vi "SETParametersToSPCdata.vi"(8 "ErrorIn":errorcluster, 10 "setFile":path=path "X:/Jannis/Abgleich/150-n scanin.set", 11 "SPCdataIn":T1={"base_adr"=0, "init"=0, "cfd_limit_low"=0.0, "cfd_limit_high"=0.0, "cfd_zc_level"=0.0, "cfd_holdoff"=0.0, "sync_zc_level"=0.0, "sync_holdoff"=0.0, "sync_threshold"=0.0, "tac_range"=0.0, "sync_freq_div"=0, "tac_gain"=0, "tac_offset"=0.0, "tac_limit_low"=0.0, "tac_limit_high"=0.0, "adc_resolution"=12, "ext_latch_delay"=0, "collect_time"=0.0, "display_time"=0.0, "repeat_time"=0.0, "stop_on_time"=0, "stop_on_ovfl"=0, "dither_range"=0, "count_incr"=0, "mem_bank"=0, "dead_time_comp"=0, "scan_control"=0, "routing_mode"=0, "tac_enable_hold"=0.0, "pci_card_no"=0, "mode"=0, "scan_size_x"=0, "scan_size_y"=0, "scan_rout_x"=0, "scan_rout_y"=0, "scan_flyback"=0, "scan_borders"=0, "scan_polarity"=0, "pixel_clock"=0, "line_compression"=0, "trigger"=0, "pixel_time"=0.0, "ext_pixclk_div"=0, "rate_count_time"=0.0, "macro_time_clk"=0, "add_select"=0, "test_eep"=0, "adc_zoom"=0, "img_size_x"=0, "img_size_y"=0, "img_rout_x"=0, "img_rout_y"=0, "xy_gain"=0, "master_clock"=0, "adc_sample_delay"=0, "detector_type"=0, "chan_enable"=0, "chan_slope"=0, "chan_spec_no"=0, "tdc_control"=0, "tdc_offset1"=0.0, "tdc_offset2"=0.0, "tdc_offset3"=0.0, "tdc_offset4"=0.0, "future_reserve1"=0, "future_reserve2"=0, "future_reserve3"=0, "future_reserve4"=0, "future_reserve5"=0, "future_reserve6"=0, "future_reserve7"=0}) -> (0 "ErrorOut":errorcluster, 3 "SPCdataOut":T1={"base_adr"=0, "init"=0, "cfd_limit_low"=0.0, "cfd_limit_high"=0.0, "cfd_zc_level"=0.0, "cfd_holdoff"=0.0, "sync_zc_level"=0.0, "sync_holdoff"=0.0, "sync_threshold"=0.0, "tac_range"=0.0, "sync_freq_div"=0, "tac_gain"=0, "tac_offset"=0.0, "tac_limit_low"=0.0, "tac_limit_high"=0.0, "adc_resolution"=12, "ext_latch_delay"=0, "collect_time"=0.0, "display_time"=0.0, "repeat_time"=0.0, "stop_on_time"=0, "stop_on_ovfl"=0, "dither_range"=0, "count_incr"=0, "mem_bank"=0, "dead_time_comp"=0, "scan_control"=0, "routing_mode"=0, "tac_enable_hold"=0.0, "pci_card_no"=0, "mode"=0, "scan_size_x"=0, "scan_size_y"=0, "scan_rout_x"=0, "scan_rout_y"=0, "scan_flyback"=0, "scan_borders"=0, "scan_polarity"=0, "pixel_clock"=0, "line_compression"=0, "trigger"=0, "pixel_time"=0.0, "ext_pixclk_div"=0, "rate_count_time"=0.0, "macro_time_clk"=0, "add_select"=0, "test_eep"=0, "adc_zoom"=0, "img_size_x"=0, "img_size_y"=0, "img_rout_x"=0, "img_rout_y"=0, "xy_gain"=0, "master_clock"=0, "adc_sample_delay"=0, "detector_type"=0, "chan_enable"=0, "chan_slope"=0, "chan_spec_no"=0, "tdc_control"=0, "tdc_offset1"=0.0, "tdc_offset2"=0.0, "tdc_offset3"=0.0, "tdc_offset4"=0.0, "future_reserve1"=0, "future_reserve2"=0, "future_reserve3"=0, "future_reserve4"=0, "future_reserve5"=0, "future_reserve6"=0, "future_reserve7"=0}, 5 "ActiveModule":string[](array[string]))   [LabVIEW 2019]
doc: "This VI aids to read a full set of system parameters from a .set-file or the header of a .sdt into the SPCdata cluster. Usefull when wanting to copy all parameters established in SPCM.exe to the LV-environment.\nNote, that some parameters like <b>mode</b> are not mapped. To correctly set these parameters use SPC_set- and get_parameters.vi before calling this VI."
uses:
  SPC_Controls/Systparm_Kewords.ctl
  SPC_Controls/SPCdata.ctl
panel:
  out "String":string
  in  "Systparm_Keywords":T2
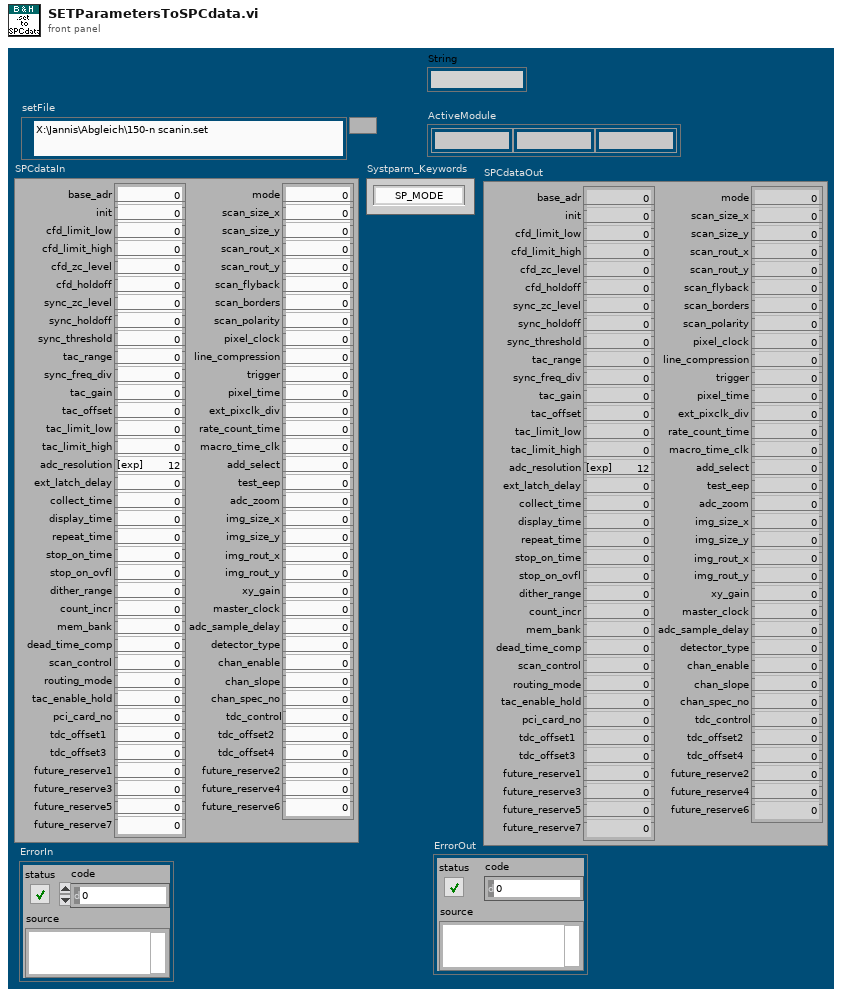
[diagram p1: front panel]
types:
  T1 = typedef "SPCdata.ctl" = cluster{"base_adr":u16, "init":i16, "cfd_limit_low":sgl, "cfd_limit_high":sgl, "cfd_zc_level":sgl, "cfd_holdoff":sgl, "sync_zc_level":sgl, "sync_holdoff":sgl, "sync_threshold":sgl, "tac_range":sgl, "sync_freq_div":i16, "tac_gain":i16, "tac_offset":sgl, "tac_limit_low":sgl, "tac_limit_high":sgl, "adc_resolution":i16, "ext_latch_delay":i16, "collect_time":sgl, "display_time":sgl, "repeat_time":sgl, "stop_on_time":i16, "stop_on_ovfl":i16, "dither_range":i16, "count_incr":i16, "mem_bank":i16, "dead_time_comp":i16, "scan_control":u16, "routing_mode":u16, "tac_enable_hold":sgl, "pci_card_no":i16, "mode":u16, "scan_size_x":u32, "scan_size_y":u32, "scan_rout_x":u32, "scan_rout_y":u32, "scan_flyback":u32, "scan_borders":u32, "scan_polarity":u16, "pixel_clock":u16, "line_compression":u16, "trigger":u16, "pixel_time":sgl, "ext_pixclk_div":u32, "rate_count_time":sgl, "macro_time_clk":i16, "add_select":i16, "test_eep":i16, "adc_zoom":i16, "img_size_x":u32, "img_size_y":u32, "img_rout_x":u32, "img_rout_y":u32, "xy_gain":i16, "master_clock":i16, "adc_sample_delay":i16, "detector_type":i16, "chan_enable":u32, "chan_slope":u32, "chan_spec_no":u32, "tdc_control":u32, "tdc_offset1":sgl, "tdc_offset2":sgl, "tdc_offset3":sgl, "tdc_offset4":sgl, "future_reserve1":u64, "future_reserve2":u64, "future_reserve3":u64, "future_reserve4":u64, "future_reserve5":u64, "future_reserve6":u64, "future_reserve7":u64}
  T2 = typedef "Systparm_Kewords.ctl" = enum16{"SP_MODE", "SP_CFD_LL", "SP_CFD_LH", "SP_CFD_ZC", "SP_CFD_HF", "SP_SYN_ZC", "SP_SYN_FD", "SP_SYN_FQ", "SP_SYN_HF", "SP_TAC_R", "SP_TAC_G", "SP_TAC_OF", "SP_TAC_LL", "SP_TAC_LH", "SP_TAC_TC", "SP_TAC_TD", "SP_ADC_RE", "SP_EAL_DE", "SP_NCX", "SP_NCY", "SP_PAGE", "SP_COL_T", "SP_REP_T", "SP_DIS_T", "SP_REPEAT", "SP_STOPT", "SP_OVERFL", "SP_WL_STA", "SP_WL_STO", "SP_WL_STE", "SP_EXTST", "SP_STEPS", "SP_OFFSET", "SP_YWIN_N", "SP_XWIN_N", "SP_TWIN_N", "SP_X_EQU", "SP_Y_EQU", "SP_T_EQU", "SP_DITH", "SP_EN_INT", "SP_INCR", "SP_DAES", "SP_SPE_FN", "SP_CYCLES", "SP_DAEC", "SP_MEM_BANK", "SP_DTCOMP", "SP_SCF", "SP_POL_L", "SP_POL_F", "SP_PIX", "SP_LDIV", "SP_ACCUM", "SP_ROUT", "SP_TAC_EH", "SP_DLIM", "SP_PHOT_F", "SP_EN_DLIM", "SP_PH_BUF", "SP_FLB_Y", "SP_FLB_X", "SP_BORD_U", "SP_BORD_L", "SP_POL_P", "SP_PIX_T", "SP_PIX_CLK", "SP_TRIGGER", "SP_SCAN_X", "SP_SCAN_Y", "SP_SCAN_RX", "SP_SCAN_RY", "SP_FIF_TYP", "SP_EPX_DIV", "SP_MTCLK", "SP_ADD_SEL", "SP_SXWIN_N", "SP_SYWIN_N", "SP_SX_EQU", "SP_SY_EQU", "SP_ASAVE", "SP_ADC_ZOOM", "SP_FIF_FNO", "SP_FCYCLES", "SP_XY_GAIN", "SP_IMG_X", "SP_IMG_Y", "SP_IMG_RX", "SP_IMG_RY", "SP_MST_CLK", "SP_ADC_DE", "SP_DET_TYP", "SP_X_AXIS", "SP_CH_EN", "SP_CH_SL", "SP_CH_F1", "SP_CH_F2"}
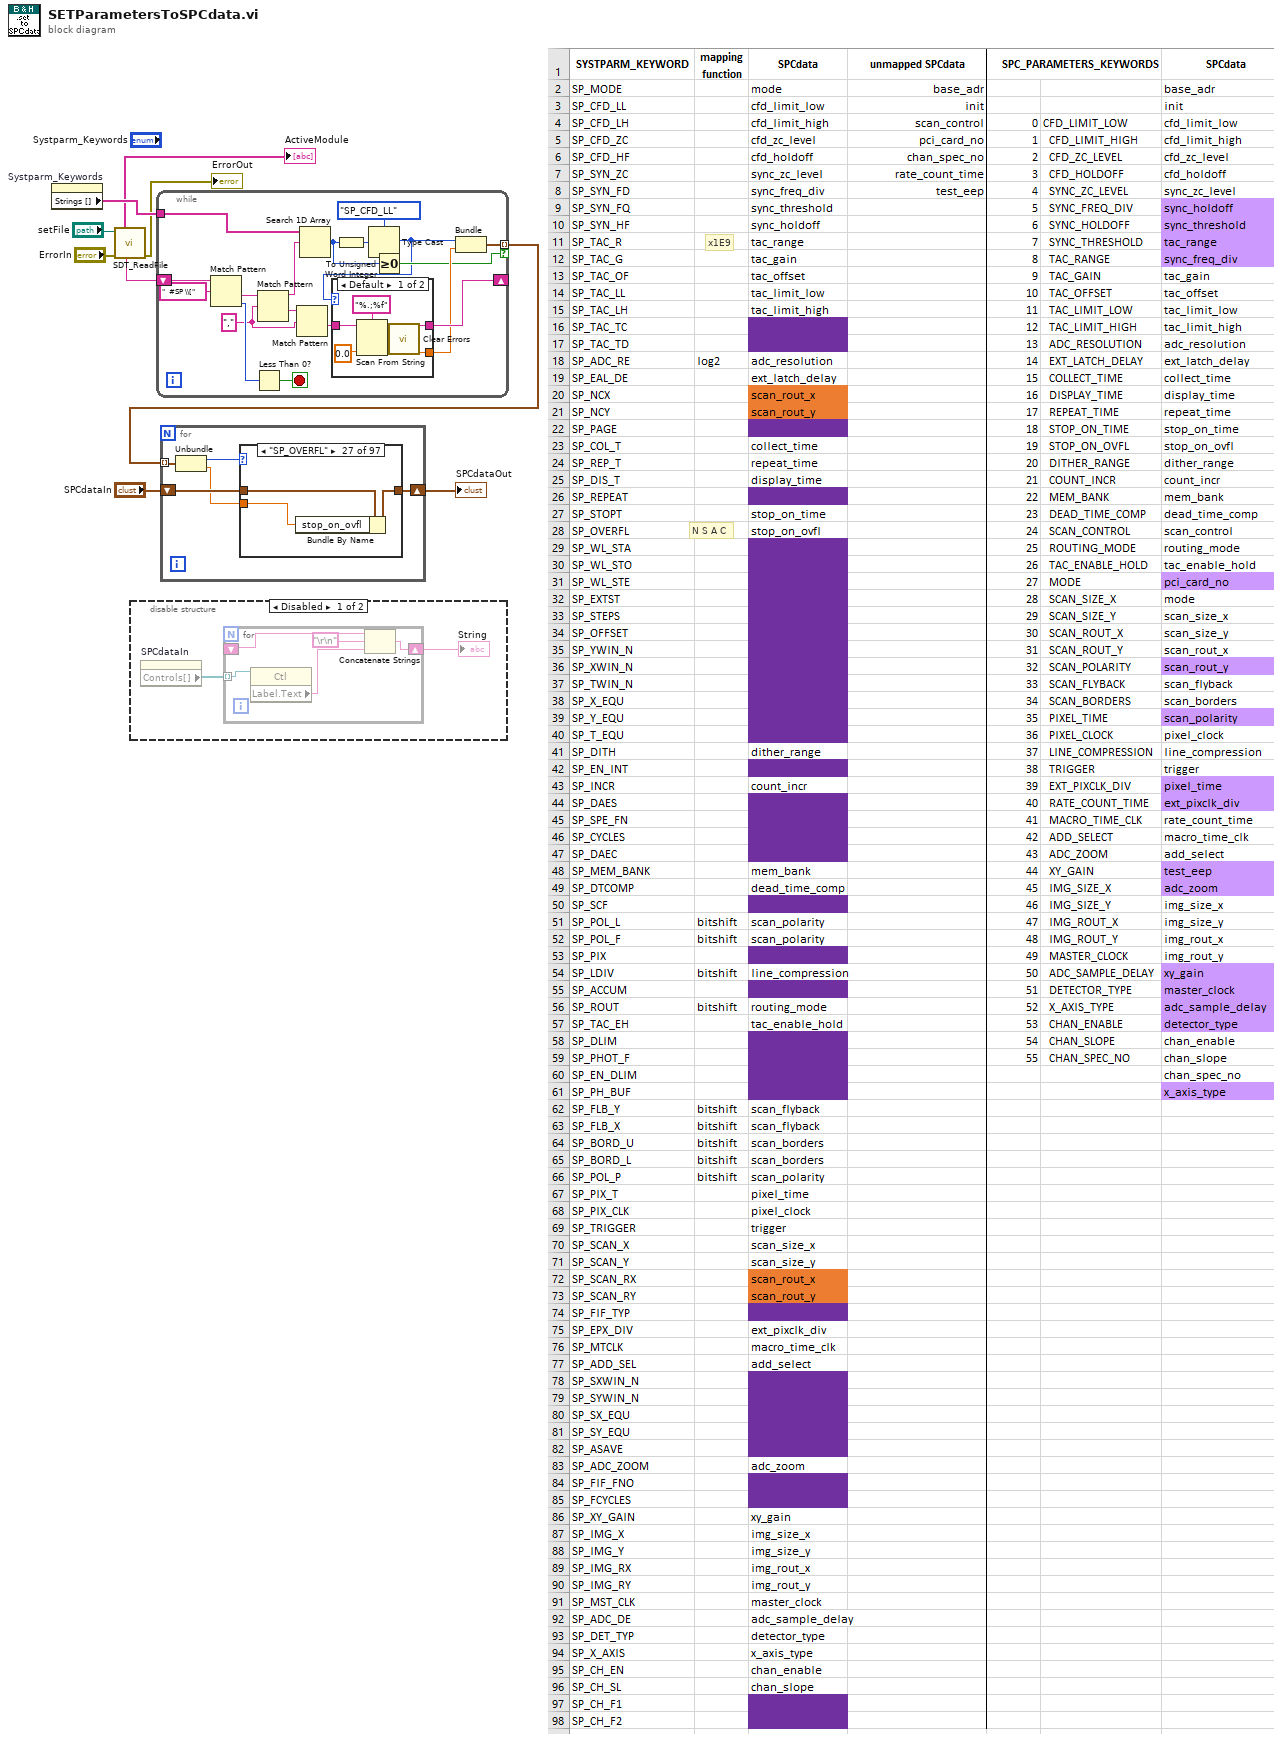
[diagram p0: block diagram]
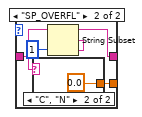
[diagram p2: hidden frame]
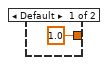
[diagram p3: hidden frame]
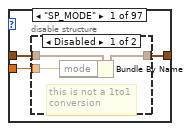
[diagram p5: hidden frame]
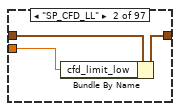
[diagram p7: hidden frame]
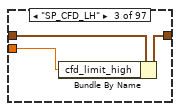
[diagram p8: hidden frame]
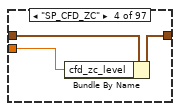
[diagram p9: hidden frame]
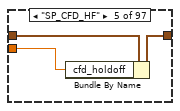
[diagram p10: hidden frame]
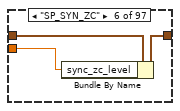
[diagram p11: hidden frame]
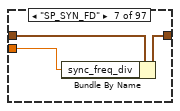
[diagram p12: hidden frame]
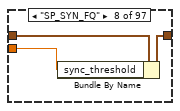
[diagram p13: hidden frame]
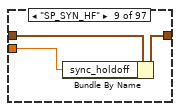
[diagram p14: hidden frame]
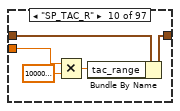
[diagram p15: hidden frame]
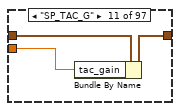
[diagram p16: hidden frame]
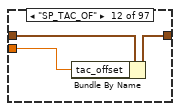
[diagram p17: hidden frame]
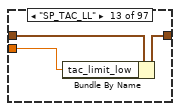
[diagram p18: hidden frame]
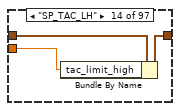
[diagram p19: hidden frame]
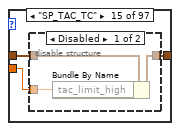
[diagram p20: hidden frame]
diagram:
  # "N S A C"
  # "x1E9"
  n1 = property on="Systparm_Keywords" class="Enum (strict)"() -> ("Strings []"=w5:string[])  [unwired: 2 in, 2 out]
  n2 = call "SDT_ReadFile.vi"("error in"="ErrorIn", "sdtFile"="setFile") -> ("error out"=→"ErrorOut":errorcluster, "SetUp"=w6:string, "ActiveModule"=→"ActiveModule":string[])  [unwired: 2 in, 5 out]
  n3 = disable-structure shown="Disabled" {
    frame Disabled {
      n4 = property on="SPCdataIn" class="Clust (strict)"() -> ("Controls[]"=w11:refnum<vi>[])  [unwired: 2 in, 2 out]
      n5 = for {
        tunnel: w11 -> [w16] mode=indexing
        shift-right: [w14] -> w10
        shift-left: _ -> [w13]
        n6 = property class="Ctl"(reference=w16) -> ("Label.Text"=w15:string)  [unwired: 1 in, 2 out]
        n7 = Concatenate Strings(w13, "\r\n", w15) -> (w14:string)
      }
      "String" <- w10
    }
    frame Enabled {
    }
  }
  n8 = while {
    shift-right: [w26] -> _
    shift-left: w6 -> [w34]
    tunnel: w5 -> [w24]
    tunnel: [w21] -> w4 mode=indexing if=w19
    stop <- w31 stop-if-true
    w28 = "," ("regular expression")
    n9 = Match Pattern(string=w34, regular expression="  #SP \\[") -> (after substring=w32:string, offset past match=w30:i32)  [unwired: 1 in, 2 out]
    n10 = Less Than 0?(x=w30) -> (x < 0?=w31:bool)
    n11 = Match Pattern(string=w32, regular expression=w28) -> (before substring=w25:string, after substring=w29:string)  [unwired: 1 in, 2 out]
    n12 = Match Pattern(string=w29, regular expression=w28) -> (after substring=w27:string)  [unwired: 1 in, 3 out]
    n13 = Search 1D Array(1D array=w24, element=w25) -> (index of element=w20:i32)  [unwired: 1 in]
    n14 = To Unsigned Word Integer(number=w20) -> (unsigned 16bit integer=w18:u16)
    n15 = Type Cast(type=Systparm_Kewords."SP_CFD_LL" ("Systparm_Keywords"), x=w18) -> (*(type *) &x=w17:T2)
    n16 = case shown="Default" w17 {
      tunnel: w27 -> [w40 w42]
      tunnel: [w37 w42] -> w26
      tunnel: [w36 w41] -> w22
      frame Default {
        n17 = Scan From String(format string="%.;%f", input string=w40, default 1=sgl 0.0 ("Value")) -> (remaining string=w37:string, error out=w35:errorcluster, output 1=w36:sgl)  [unwired: 2 in, 1 out]
        n18 = call <vilib>:"Clear Errors.vi"("error in (no error)"=w35) -> ()  [unwired: 5 in, 2 out]
      }
      frame "SP_OVERFL" {
        n19 = String Subset(string=w42, length (rest)=1 ("length (rest)")) -> (substring=w43:string)  [unwired: 1 in]
        n20 = case shown="\"C\", \"N\"" w43 {
          tunnel: [sgl 1.0 ("Value") sgl 0.0 ("Value")] -> w41
          frame Default {
          }
          frame "C", "N" {
          }
        }
      }
    }
    n21 = Greater Or Equal To 0?(x=w20) -> (x >= 0?=w19:bool)
    n22 = Bundle("Systparm_Keywords"=w17, "Value"=w22) -> (w21:cluster{"Systparm_Keywords":T2, "Value":sgl})  [unwired: 1 in]
  }
  n23 = for {
    shift-right: [w50] -> w8
    shift-left: "SPCdataIn" -> [w51]
    tunnel: w4 -> [w49] mode=indexing
    n24 = Unbundle(w49) -> ("Systparm_Keywords"=w48:T2, "Value"=w47:sgl)
    n25 = case shown="\"SP_OVERFL\"" w48 {
      tunnel: w51 -> [w53 w61 w64 w67 w70 w73 w76 w79 w82 w87 w90 w93 w96 w99 w102 w109 w117 w120 w123 w126 w129 w136 w139 w142 w145 w152 w155 w158 w165 w172 w179 w186 w193 w200 w207 w214 w221 w228 w235 w242 w245 w252 w255 w262 w269 w276 w283 w286 w289 w300 w310 w314 w323 w326 w335 w338 w341 w348 w355 w362 w374 w381 w390 w397 w407 w410 w413 w416 w419 w422 w425 w428 w431 w438 w441 w444 w447 w454 w461 w468 w475 w482 w485 w492 w499 w502 w505 w508 w511 w514 w517 w520 w523 w526 w529 w532 w539]
      tunnel: [w54 w60 w63 w66 w69 w72 w75 w78 w81 w86 w89 w92 w95 w98 w101 w108 w116 w119 w122 w125 w128 w135 w138 w141 w144 w151 w154 w157 w164 w171 w178 w185 w192 w199 w206 w213 w220 w227 w234 w241 w244 w251 w254 w261 w268 w275 w282 w285 w288 w301 w311 w313 w322 w325 w334 w337 w340 w347 w354 w361 w375 w382 w391 w398 w408 w411 w414 w417 w420 w423 w426 w429 w432 w439 w442 w445 w448 w455 w462 w469 w476 w483 w486 w493 w500 w503 w506 w509 w512 w515 w518 w521 w524 w527 w530 w533 w540] -> w50
      tunnel: w47 -> [w52 w59 w62 w65 w68 w71 w74 w77 w80 w85 w88 w91 w94 w97 w100 w107 w115 w118 w121 w124 w127 w134 w137 w140 w143 w150 w153 w156 w163 w170 w177 w184 w191 w198 w205 w212 w219 w226 w233 w240 w243 w250 w253 w260 w267 w274 w281 w284 w287 w297 w305 w312 w321 w324 w333 w336 w339 w346 w353 w360 w371 w376 w385 w392 w402 w409 w412 w415 w418 w421 w424 w427 w430 w437 w440 w443 w446 w453 w460 w467 w474 w481 w484 w491 w498 w501 w504 w507 w510 w513 w516 w519 w522 w525 w528 w531 w538]
      frame "SP_MODE" {
        n26 = disable-structure shown="Disabled" {
          disable-tunnel: [w57 w58] -> w54
          disable-tunnel: w53 -> [w56 w58]
          disable-tunnel: w52 -> [w55 _]
          frame Disabled {
            # "this is not a 1to1\nconversion"
            n27 = Bundle By Name(cluster=w56, "mode"=w55) -> (w57:T1)
          }
          frame Enabled {
          }
        }
      }
      frame "SP_CFD_LL" {
        n28 = Bundle By Name(cluster=w61, "cfd_limit_low"=w59) -> (w60:T1)
      }
      frame "SP_CFD_LH" {
        n29 = Bundle By Name(cluster=w64, "cfd_limit_high"=w62) -> (w63:T1)
      }
      frame "SP_CFD_ZC" {
        n30 = Bundle By Name(cluster=w67, "cfd_zc_level"=w65) -> (w66:T1)
      }
      frame "SP_CFD_HF" {
        n31 = Bundle By Name(cluster=w70, "cfd_holdoff"=w68) -> (w69:T1)
      }
      frame "SP_SYN_ZC" {
        n32 = Bundle By Name(cluster=w73, "sync_zc_level"=w71) -> (w72:T1)
      }
      frame "SP_SYN_FD" {
        n33 = Bundle By Name(cluster=w76, "sync_freq_div"=w74) -> (w75:T1)
      }
      frame "SP_SYN_FQ" {
        n34 = Bundle By Name(cluster=w79, "sync_threshold"=w77) -> (w78:T1)
      }
      frame "SP_SYN_HF" {
        n35 = Bundle By Name(cluster=w82, "sync_holdoff"=w80) -> (w81:T1)
      }
      frame "SP_TAC_R" {
        n36 = Multiply(x=w85, y=sgl 1000000000.0) -> (x*y=w84:sgl)
        n37 = Bundle By Name(cluster=w87, "tac_range"=w84) -> (w86:T1)
      }
      frame "SP_TAC_G" {
        n38 = Bundle By Name(cluster=w90, "tac_gain"=w88) -> (w89:T1)
      }
      frame "SP_TAC_OF" {
        n39 = Bundle By Name(cluster=w93, "tac_offset"=w91) -> (w92:T1)
      }
      frame "SP_TAC_LL" {
        n40 = Bundle By Name(cluster=w96, "tac_limit_low"=w94) -> (w95:T1)
      }
      frame "SP_TAC_LH" {
        n41 = Bundle By Name(cluster=w99, "tac_limit_high"=w97) -> (w98:T1)
      }
      frame "SP_TAC_TC" {
        n42 = disable-structure shown="Disabled" {
          disable-tunnel: w102 -> [w105 w106]
          disable-tunnel: [w104 w106] -> w101
          disable-tunnel: w100 -> [w103 _]
          frame Disabled {
            n43 = Bundle By Name(cluster=w105, "tac_limit_high"=w103) -> (w104:T1)
          }
          frame Enabled {
          }
        }
      }
      frame "SP_TAC_TD" {
        n44 = disable-structure shown="Enabled" {
          disable-tunnel: w109 -> [w112 w113]
          disable-tunnel: [w111 w113] -> w108
          disable-tunnel: w107 -> [w110 _]
          frame Disabled {
            n45 = Bundle By Name(cluster=w112, "sync_holdoff"=w110) -> (w111:T1)
          }
          frame Enabled {
          }
        }
      }
      frame "SP_ADC_RE" {
        n46 = Logarithm Base 2(1:w115) -> (0:w114:sgl)
        n47 = Bundle By Name(cluster=w117, "adc_resolution"=w114) -> (w116:T1)
      }
      frame "SP_EAL_DE" {
        n48 = Bundle By Name(cluster=w120, "ext_latch_delay"=w118) -> (w119:T1)
      }
      frame "SP_NCX" {
        n49 = Bundle By Name(cluster=w123, "scan_rout_x"=w121) -> (w122:T1)
      }
      frame "SP_NCY" {
        n50 = Bundle By Name(cluster=w126, "scan_rout_y"=w124) -> (w125:T1)
      }
      frame "SP_PAGE" {
        n51 = disable-structure shown="Disabled" {
          disable-tunnel: w129 -> [w132 w133]
          disable-tunnel: [w131 w133] -> w128
          disable-tunnel: w127 -> [w130 _]
          frame Disabled {
            n52 = Bundle By Name(cluster=w132, "scan_rout_y"=w130) -> (w131:T1)
          }
          frame Enabled {
          }
        }
      }
      frame "SP_COL_T" {
        n53 = Bundle By Name(cluster=w136, "collect_time"=w134) -> (w135:T1)
      }
      frame "SP_REP_T" {
        n54 = Bundle By Name(cluster=w139, "repeat_time"=w137) -> (w138:T1)
      }
      frame "SP_DIS_T" {
        n55 = Bundle By Name(cluster=w142, "display_time"=w140) -> (w141:T1)
      }
      frame "SP_REPEAT" {
        n56 = disable-structure shown="Disabled" {
          disable-tunnel: w145 -> [w148 w149]
          disable-tunnel: [w147 w149] -> w144
          disable-tunnel: w143 -> [w146 _]
          frame Disabled {
            n57 = Bundle By Name(cluster=w148, "repeat_time"=w146) -> (w147:T1)
          }
          frame Enabled {
          }
        }
      }
      frame "SP_STOPT" {
        n58 = Bundle By Name(cluster=w152, "stop_on_time"=w150) -> (w151:T1)
      }
      frame "SP_OVERFL" {
        n59 = Bundle By Name(cluster=w155, "stop_on_ovfl"=w153) -> (w154:T1)
      }
      frame "SP_WL_STA" {
        n60 = disable-structure shown="Disabled" {
          disable-tunnel: w158 -> [w161 w162]
          disable-tunnel: [w160 w162] -> w157
          disable-tunnel: w156 -> [w159 _]
          frame Disabled {
            n61 = Bundle By Name(cluster=w161, "stop_on_ovfl"=w159) -> (w160:T1)
          }
          frame Enabled {
          }
        }
      }
      frame "SP_WL_STO" {
        n62 = disable-structure shown="Disabled" {
          disable-tunnel: w165 -> [w168 w169]
          disable-tunnel: [w167 w169] -> w164
          disable-tunnel: w163 -> [w166 _]
          frame Disabled {
            n63 = Bundle By Name(cluster=w168, "stop_on_ovfl"=w166) -> (w167:T1)
          }
          frame Enabled {
          }
        }
      }
      frame "SP_WL_STE" {
        n64 = disable-structure shown="Disabled" {
          disable-tunnel: w172 -> [w175 w176]
          disable-tunnel: [w174 w176] -> w171
          disable-tunnel: w170 -> [w173 _]
          frame Disabled {
            n65 = Bundle By Name(cluster=w175, "stop_on_ovfl"=w173) -> (w174:T1)
          }
          frame Enabled {
          }
        }
      }
      frame "SP_EXTST" {
        n66 = disable-structure shown="Disabled" {
          disable-tunnel: w179 -> [w182 w183]
          disable-tunnel: [w181 w183] -> w178
          disable-tunnel: w177 -> [w180 _]
          frame Disabled {
            n67 = Bundle By Name(cluster=w182, "stop_on_ovfl"=w180) -> (w181:T1)
          }
          frame Enabled {
          }
        }
      }
      frame "SP_STEPS" {
        n68 = disable-structure shown="Disabled" {
          disable-tunnel: w186 -> [w189 w190]
          disable-tunnel: [w188 w190] -> w185
          disable-tunnel: w184 -> [w187 _]
          frame Disabled {
            n69 = Bundle By Name(cluster=w189, "stop_on_ovfl"=w187) -> (w188:T1)
          }
          frame Enabled {
          }
        }
      }
      frame "SP_OFFSET" {
        n70 = disable-structure shown="Disabled" {
          disable-tunnel: w193 -> [w196 w197]
          disable-tunnel: [w195 w197] -> w192
          disable-tunnel: w191 -> [w194 _]
          frame Disabled {
            n71 = Bundle By Name(cluster=w196, "stop_on_ovfl"=w194) -> (w195:T1)
          }
          frame Enabled {
          }
        }
      }
      frame "SP_YWIN_N" {
        n72 = disable-structure shown="Disabled" {
          disable-tunnel: w200 -> [w203 w204]
          disable-tunnel: [w202 w204] -> w199
          disable-tunnel: w198 -> [w201 _]
          frame Disabled {
            n73 = Bundle By Name(cluster=w203, "stop_on_ovfl"=w201) -> (w202:T1)
          }
          frame Enabled {
          }
        }
      }
      frame "SP_XWIN_N" {
        n74 = disable-structure shown="Disabled" {
          disable-tunnel: w207 -> [w210 w211]
          disable-tunnel: [w209 w211] -> w206
          disable-tunnel: w205 -> [w208 _]
          frame Disabled {
            n75 = Bundle By Name(cluster=w210, "stop_on_ovfl"=w208) -> (w209:T1)
          }
          frame Enabled {
          }
        }
      }
      frame "SP_TWIN_N" {
        n76 = disable-structure shown="Disabled" {
          disable-tunnel: w214 -> [w217 w218]
          disable-tunnel: [w216 w218] -> w213
          disable-tunnel: w212 -> [w215 _]
          frame Disabled {
            n77 = Bundle By Name(cluster=w217, "stop_on_ovfl"=w215) -> (w216:T1)
          }
          frame Enabled {
          }
        }
      }
      frame "SP_X_EQU" {
        n78 = disable-structure shown="Disabled" {
          disable-tunnel: w221 -> [w224 w225]
          disable-tunnel: [w223 w225] -> w220
          disable-tunnel: w219 -> [w222 _]
          frame Disabled {
            n79 = Bundle By Name(cluster=w224, "stop_on_ovfl"=w222) -> (w223:T1)
          }
          frame Enabled {
          }
        }
      }
      frame "SP_Y_EQU" {
        n80 = disable-structure shown="Disabled" {
          disable-tunnel: w228 -> [w231 w232]
          disable-tunnel: [w230 w232] -> w227
          disable-tunnel: w226 -> [w229 _]
          frame Disabled {
            n81 = Bundle By Name(cluster=w231, "stop_on_ovfl"=w229) -> (w230:T1)
          }
          frame Enabled {
          }
        }
      }
      frame "SP_T_EQU" {
        n82 = disable-structure shown="Disabled" {
          disable-tunnel: w235 -> [w238 w239]
          disable-tunnel: [w237 w239] -> w234
          disable-tunnel: w233 -> [w236 _]
          frame Disabled {
            n83 = Bundle By Name(cluster=w238, "stop_on_ovfl"=w236) -> (w237:T1)
          }
          frame Enabled {
          }
        }
      }
      frame "SP_DITH" {
        n84 = Bundle By Name(cluster=w242, "dither_range"=w240) -> (w241:T1)
      }
      frame "SP_EN_INT" {
        n85 = disable-structure shown="Disabled" {
          disable-tunnel: w245 -> [w248 w249]
          disable-tunnel: [w247 w249] -> w244
          disable-tunnel: w243 -> [w246 _]
          frame Disabled {
            n86 = Bundle By Name(cluster=w248, "dither_range"=w246) -> (w247:T1)
          }
          frame Enabled {
          }
        }
      }
      frame "SP_INCR" {
        n87 = Bundle By Name(cluster=w252, "count_incr"=w250) -> (w251:T1)
      }
      frame "SP_DAES" {
        n88 = disable-structure shown="Disabled" {
          disable-tunnel: w255 -> [w258 w259]
          disable-tunnel: [w257 w259] -> w254
          disable-tunnel: w253 -> [w256 _]
          frame Disabled {
            n89 = Bundle By Name(cluster=w258, "count_incr"=w256) -> (w257:T1)
          }
          frame Enabled {
          }
        }
      }
      frame "SP_SPE_FN" {
        n90 = disable-structure shown="Disabled" {
          disable-tunnel: w262 -> [w265 w266]
          disable-tunnel: [w264 w266] -> w261
          disable-tunnel: w260 -> [w263 _]
          frame Disabled {
            n91 = Bundle By Name(cluster=w265, "count_incr"=w263) -> (w264:T1)
          }
          frame Enabled {
          }
        }
      }
      frame "SP_CYCLES" {
        n92 = disable-structure shown="Disabled" {
          disable-tunnel: w269 -> [w272 w273]
          disable-tunnel: [w271 w273] -> w268
          disable-tunnel: w267 -> [w270 _]
          frame Disabled {
            n93 = Bundle By Name(cluster=w272, "count_incr"=w270) -> (w271:T1)
          }
          frame Enabled {
          }
        }
      }
      frame "SP_DAEC" {
        n94 = disable-structure shown="Disabled" {
          disable-tunnel: w276 -> [w279 w280]
          disable-tunnel: [w278 w280] -> w275
          disable-tunnel: w274 -> [w277 _]
          frame Disabled {
            n95 = Bundle By Name(cluster=w279, "count_incr"=w277) -> (w278:T1)
          }
          frame Enabled {
          }
        }
      }
      frame "SP_MEM_BANK" {
        n96 = Bundle By Name(cluster=w283, "mem_bank"=w281) -> (w282:T1)
      }
      frame "SP_DTCOMP" {
        n97 = Bundle By Name(cluster=w286, "dead_time_comp"=w284) -> (w285:T1)
      }
      frame "SP_SCF" {
        n98 = disable-structure shown="Disabled" {
          disable-tunnel: w289 -> [w292 w293]
          disable-tunnel: [w291 w293] -> w288
          disable-tunnel: w287 -> [w290 _]
          frame Disabled {
            n99 = Bundle By Name(cluster=w292, "mem_bank"=w290) -> (w291:T1)
          }
          frame Enabled {
          }
        }
      }
      frame "SP_POL_L" {
        n100 = To Unsigned Word Integer(number=w297) -> (unsigned 16bit integer=w294:u16)
        n101 = Unbundle By Name(w300) -> ("scan_polarity"=w299:u16)
        n102 = And(x=w299, y=u16 65534) -> (x .and. y?=w295:u16)
        n103 = Or(x=w295, y=w294) -> (x .or. y?=w296:u16)
        n104 = Bundle By Name(cluster=w300, "scan_polarity"=w296) -> (w301:T1)
      }
      frame "SP_POL_F" {
        n105 = To Unsigned Word Integer(number=w305) -> (unsigned 16bit integer=w302:u16)
        n106 = Unbundle By Name(w310) -> ("scan_polarity"=w309:u16)
        n107 = Logical Shift(y=u16 1 ("x .and. y?"), x=w302) -> (x << y=w304:u16)
        n108 = And(x=w309, y=u16 65533) -> (x .and. y?=w306:u16)
        n109 = Or(x=w306, y=w304) -> (x .or. y?=w307:u16)
        n110 = Bundle By Name(cluster=w310, "scan_polarity"=w307) -> (w311:T1)
      }
      frame "SP_PIX" {
        n111 = disable-structure shown="Disabled" {
          disable-tunnel: w314 -> [w317 w318]
          disable-tunnel: [w316 w318] -> w313
          disable-tunnel: w312 -> [w315 _]
          frame Disabled {
            n112 = Bundle By Name(cluster=w317, "mem_bank"=w315) -> (w316:T1)
          }
          frame Enabled {
          }
        }
      }
      frame "SP_LDIV" {
        n113 = Logical Shift(y=w321, x=i16 1 ("y")) -> (x << y=w320:i16)
        n114 = Bundle By Name(cluster=w323, "line_compression"=w320) -> (w322:T1)
      }
      frame "SP_ACCUM" {
        n115 = disable-structure shown="Disabled" {
          disable-tunnel: w326 -> [w329 w330]
          disable-tunnel: [w328 w330] -> w325
          disable-tunnel: w324 -> [w327 _]
          frame Disabled {
            n116 = Bundle By Name(cluster=w329, "pixel_clock"=w327) -> (w328:T1)
          }
          frame Enabled {
          }
        }
      }
      frame "SP_ROUT" {
        n117 = Logical Shift(y=i16 6, x=w333) -> (x << y=w332:u32)
        n118 = Bundle By Name(cluster=w335, "routing_mode"=w332) -> (w334:T1)
      }
      frame "SP_TAC_EH" {
        n119 = Bundle By Name(cluster=w338, "tac_enable_hold"=w336) -> (w337:T1)
      }
      frame "SP_DLIM" {
        n120 = disable-structure shown="Disabled" {
          disable-tunnel: w341 -> [w344 w345]
          disable-tunnel: [w343 w345] -> w340
          disable-tunnel: w339 -> [w342 _]
          frame Disabled {
            n121 = Bundle By Name(cluster=w344, "tac_enable_hold"=w342) -> (w343:T1)
          }
          frame Enabled {
          }
        }
      }
      frame "SP_PHOT_F" {
        n122 = disable-structure shown="Disabled" {
          disable-tunnel: w348 -> [w351 w352]
          disable-tunnel: [w350 w352] -> w347
          disable-tunnel: w346 -> [w349 _]
          frame Disabled {
            n123 = Bundle By Name(cluster=w351, "tac_enable_hold"=w349) -> (w350:T1)
          }
          frame Enabled {
          }
        }
      }
      frame "SP_EN_DLIM" {
        n124 = disable-structure shown="Disabled" {
          disable-tunnel: w355 -> [w358 w359]
          disable-tunnel: [w357 w359] -> w354
          disable-tunnel: w353 -> [w356 _]
          frame Disabled {
            n125 = Bundle By Name(cluster=w358, "tac_enable_hold"=w356) -> (w357:T1)
          }
          frame Enabled {
          }
        }
      }
      frame "SP_PH_BUF" {
        n126 = disable-structure shown="Disabled" {
          disable-tunnel: w362 -> [w365 w366]
          disable-tunnel: [w364 w366] -> w361
          disable-tunnel: w360 -> [w363 _]
          frame Disabled {
            n127 = Bundle By Name(cluster=w365, "tac_enable_hold"=w363) -> (w364:T1)
          }
          frame Enabled {
          }
        }
      }
      frame "SP_FLB_Y" {
        n128 = Unbundle By Name(w374) -> ("scan_flyback"=w373:u32)
        n129 = Logical Shift(y=i16 16, x=w371) -> (x << y=w369:u32)
        n130 = And(x=w373, y=u32 65535) -> (x .and. y?=w367:u32)
        n131 = Or(x=w367, y=w369) -> (x .or. y?=w368:u32)
        n132 = Bundle By Name(cluster=w374, "scan_flyback"=w368) -> (w375:T1)
      }
      frame "SP_FLB_X" {
        n133 = Unbundle By Name(w381) -> ("scan_flyback"=w380:u32)
        n134 = And(x=w380, y=u32 4294901760) -> (x .and. y?=w377:u32)
        n135 = Or(x=w377, y=w376) -> (x .or. y?=w378:i32)
        n136 = Bundle By Name(cluster=w381, "scan_flyback"=w378) -> (w382:T1)
      }
      frame "SP_BORD_U" {
        n137 = Unbundle By Name(w390) -> ("scan_borders"=w389:u32)
        n138 = Logical Shift(y=i16 16, x=w385) -> (x << y=w384:u32)
        n139 = And(x=w389, y=u32 65535) -> (x .and. y?=w386:u32)
        n140 = Or(x=w386, y=w384) -> (x .or. y?=w387:u32)
        n141 = Bundle By Name(cluster=w390, "scan_borders"=w387) -> (w391:T1)
      }
      frame "SP_BORD_L" {
        n142 = Unbundle By Name(w397) -> ("scan_borders"=w396:u32)
        n143 = And(x=w396, y=u32 4294901760) -> (x .and. y?=w393:u32)
        n144 = Or(x=w393, y=w392) -> (x .or. y?=w394:i32)
        n145 = Bundle By Name(cluster=w397, "scan_borders"=w394) -> (w398:T1)
      }
      frame "SP_POL_P" {
        n146 = To Unsigned Word Integer(number=w402) -> (unsigned 16bit integer=w399:u16)
        n147 = Unbundle By Name(w407) -> ("scan_polarity"=w406:u16)
        n148 = Logical Shift(y=i16 2, x=w399) -> (x << y=w401:u16)
        n149 = And(x=w406, y=u16 65531) -> (x .and. y?=w403:u16)
        n150 = Or(x=w403, y=w401) -> (x .or. y?=w404:u16)
        n151 = Bundle By Name(cluster=w407, "scan_polarity"=w404) -> (w408:T1)
      }
      frame "SP_PIX_T" {
        n152 = Bundle By Name(cluster=w410, "pixel_time"=w409) -> (w411:T1)
      }
      frame "SP_PIX_CLK" {
        n153 = Bundle By Name(cluster=w413, "pixel_clock"=w412) -> (w414:T1)
      }
      frame "SP_TRIGGER" {
        n154 = Bundle By Name(cluster=w416, "trigger"=w415) -> (w417:T1)
      }
      frame "SP_SCAN_X" {
        n155 = Bundle By Name(cluster=w419, "scan_size_x"=w418) -> (w420:T1)
      }
      frame "SP_SCAN_Y" {
        n156 = Bundle By Name(cluster=w422, "scan_size_y"=w421) -> (w423:T1)
      }
      frame "SP_SCAN_RX" {
        n157 = Bundle By Name(cluster=w425, "scan_rout_x"=w424) -> (w426:T1)
      }
      frame "SP_SCAN_RY" {
        n158 = Bundle By Name(cluster=w428, "scan_rout_y"=w427) -> (w429:T1)
      }
      frame "SP_FIF_TYP" {
        n159 = disable-structure shown="Disabled" {
          disable-tunnel: [w435 w436] -> w432
          disable-tunnel: w431 -> [w434 w436]
          disable-tunnel: w430 -> [w433 _]
          frame Disabled {
            n160 = Bundle By Name(cluster=w434, "scan_rout_y"=w433) -> (w435:T1)
          }
          frame Enabled {
          }
        }
      }
      frame "SP_EPX_DIV" {
        n161 = Bundle By Name(cluster=w438, "ext_pixclk_div"=w437) -> (w439:T1)
      }
      frame "SP_MTCLK" {
        n162 = Bundle By Name(cluster=w441, "macro_time_clk"=w440) -> (w442:T1)
      }
      frame "SP_ADD_SEL" {
        n163 = Bundle By Name(cluster=w444, "add_select"=w443) -> (w445:T1)
      }
      frame "SP_SXWIN_N" {
        n164 = disable-structure shown="Disabled" {
          disable-tunnel: [w451 w452] -> w448
          disable-tunnel: w447 -> [w450 w452]
          disable-tunnel: w446 -> [w449 _]
          frame Disabled {
            n165 = Bundle By Name(cluster=w450, "add_select"=w449) -> (w451:T1)
          }
          frame Enabled {
          }
        }
      }
      frame "SP_SYWIN_N" {
        n166 = disable-structure shown="Disabled" {
          disable-tunnel: [w458 w459] -> w455
          disable-tunnel: w454 -> [w457 w459]
          disable-tunnel: w453 -> [w456 _]
          frame Disabled {
            n167 = Bundle By Name(cluster=w457, "add_select"=w456) -> (w458:T1)
          }
          frame Enabled {
          }
        }
      }
      frame "SP_SX_EQU" {
        n168 = disable-structure shown="Disabled" {
          disable-tunnel: [w465 w466] -> w462
          disable-tunnel: w461 -> [w464 w466]
          disable-tunnel: w460 -> [w463 _]
          frame Disabled {
            n169 = Bundle By Name(cluster=w464, "add_select"=w463) -> (w465:T1)
          }
          frame Enabled {
          }
        }
      }
      frame "SP_SY_EQU" {
        n170 = disable-structure shown="Disabled" {
          disable-tunnel: [w472 w473] -> w469
          disable-tunnel: w468 -> [w471 w473]
          disable-tunnel: w467 -> [w470 _]
          frame Disabled {
            n171 = Bundle By Name(cluster=w471, "add_select"=w470) -> (w472:T1)
          }
          frame Enabled {
          }
        }
      }
      frame "SP_ASAVE" {
        n172 = disable-structure shown="Disabled" {
          disable-tunnel: [w479 w480] -> w476
          disable-tunnel: w475 -> [w478 w480]
          disable-tunnel: w474 -> [w477 _]
          frame Disabled {
            n173 = Bundle By Name(cluster=w478, "add_select"=w477) -> (w479:T1)
          }
          frame Enabled {
          }
        }
      }
      frame "SP_ADC_ZOOM" {
        n174 = Bundle By Name(cluster=w482, "adc_zoom"=w481) -> (w483:T1)
      }
      frame "SP_FIF_FNO" {
        n175 = disable-structure shown="Disabled" {
          disable-tunnel: [w489 w490] -> w486
          disable-tunnel: w485 -> [w488 w490]
          disable-tunnel: w484 -> [w487 _]
          frame Disabled {
            n176 = Bundle By Name(cluster=w488, "adc_zoom"=w487) -> (w489:T1)
          }
          frame Enabled {
          }
        }
      }
      frame "SP_FCYCLES" {
        n177 = disable-structure shown="Disabled" {
          disable-tunnel: [w496 w497] -> w493
          disable-tunnel: w492 -> [w495 w497]
          disable-tunnel: w491 -> [w494 _]
          frame Disabled {
            n178 = Bundle By Name(cluster=w495, "adc_zoom"=w494) -> (w496:T1)
          }
          frame Enabled {
          }
        }
      }
      frame "SP_XY_GAIN" {
        n179 = Bundle By Name(cluster=w499, "xy_gain"=w498) -> (w500:T1)
      }
      frame "SP_IMG_X" {
        n180 = Bundle By Name(cluster=w502, "img_size_x"=w501) -> (w503:T1)
      }
      frame "SP_IMG_Y" {
        n181 = Bundle By Name(cluster=w505, "img_size_y"=w504) -> (w506:T1)
      }
      frame "SP_IMG_RX" {
        n182 = Bundle By Name(cluster=w508, "img_rout_x"=w507) -> (w509:T1)
      }
      frame "SP_IMG_RY" {
        n183 = Bundle By Name(cluster=w511, "img_rout_y"=w510) -> (w512:T1)
      }
      frame "SP_MST_CLK" {
        n184 = Bundle By Name(cluster=w514, "master_clock"=w513) -> (w515:T1)
      }
      frame "SP_ADC_DE" {
        n185 = Bundle By Name(cluster=w517, "adc_sample_delay"=w516) -> (w518:T1)
      }
      frame "SP_DET_TYP" {
        n186 = Bundle By Name(cluster=w520, "detector_type"=w519) -> (w521:T1)
      }
      frame "SP_X_AXIS" {
        n187 = Bundle By Name(cluster=w523, "tdc_control"=w522) -> (w524:T1)
      }
      frame "SP_CH_EN" {
        n188 = Bundle By Name(cluster=w526, "chan_enable"=w525) -> (w527:T1)
      }
      frame "SP_CH_SL" {
        n189 = Bundle By Name(cluster=w529, "chan_slope"=w528) -> (w530:T1)
      }
      frame "SP_CH_F1" {
        n190 = disable-structure shown="Enabled" {
          disable-tunnel: [w536 w537] -> w533
          disable-tunnel: w532 -> [w535 w537]
          disable-tunnel: w531 -> [w534 _]
          frame Disabled {
            n191 = Bundle By Name(cluster=w535, "chan_slope"=w534) -> (w536:T1)
          }
          frame Enabled {
          }
        }
      }
      frame "SP_CH_F2" {
        n192 = disable-structure shown="Disabled" {
          disable-tunnel: [w543 w544] -> w540
          disable-tunnel: w539 -> [w542 w544]
          disable-tunnel: w538 -> [w541 _]
          frame Disabled {
            n193 = Bundle By Name(cluster=w542, "chan_slope"=w541) -> (w543:T1)
          }
          frame Enabled {
          }
        }
      }
    }
  }
  "SPCdataOut" <- w8
